vi "Init Array of VacuumLine Config Objs.vi"(8 "error in (no error)":errorcluster, 11 "VacuumLines Configuration in":refnum<class "VacuumLines Configuration.lvclass">) -> (0 "error out":errorcluster, 2 "Array of VacuumLine Config Objs":refnum<class "VacuumLine Configuration.lvclass">[](array[class]), 3 "VacuumLines Configuration out":refnum<class "VacuumLines Configuration.lvclass">)   [LabVIEW 2016, in "Hardware.lvlib" / "VacuumLine.lvlib" / "VacuumLines Configuration.lvclass"]
uses:
  <userlib>/Common Components/Hardware/Abstract System/VacuumLine/VacuumLines Configuration/VacuumLines Configuration.lvclass
  C:/Program Files (x86)/National Instruments/LabVIEW 2016/user.lib/Configuration Dialog Actor/Configuration.lvclass
  <userlib>/Common Components/Hardware/Abstract System/VacuumLine/VacuumLine Config/VacuumLine Configuration.lvclass
  <userlib>/Common Components/Hardware/Abstract System/VacuumLine/VacuumLines Configuration/VacuumLines Configuration.lvclass/VacuumLines Configuration.ctl
  <userlib>/Configuration Dialog Actor/Configuration.lvclass/Configuration.ctl
  <userlib>/Common Components/Hardware/Abstract System/VacuumLine/VacuumLines/VacuumLines.lvclass/VacuumLines.ctl
  <userlib>/Common Components/Hardware/Abstract System/VacuumLine/VacuumLine Config/VacuumLine Configuration.lvclass/VacuumLine Configuration.ctl
  <userlib>/Common Components/Hardware/Abstract System/VacuumLine/VacuumLine Config/Accessors/Write VacuumLine Obj.vi
  <userlib>/Configuration Dialog Actor/Accessors/Write Change Display.vi
  <userlib>/Configuration Dialog Actor/Accessors/Write Sub Panel.vi
  <userlib>/Configuration Dialog Actor/Accessors/Write Title.vi
  <userlib>/Configuration Dialog Actor/Accessors/Write Categories.vi
  <userlib>/Common Components/Hardware/Abstract System/VacuumLine/VacuumLines Configuration/Accessors/Read VacuumLines Obj.vi
  <userlib>/Configuration Dialog Actor/Accessors/Read Change Display.vi
  <userlib>/Configuration Dialog Actor/Accessors/Read Sub Panel.vi
  <userlib>/Configuration Dialog Actor/Accessors/Read Title.vi
  <userlib>/Configuration Dialog Actor/Accessors/Read Categories.vi
  <userlib>/Common Components/Hardware/Abstract System/VacuumLine/VacuumLines/VacuumLines.lvclass
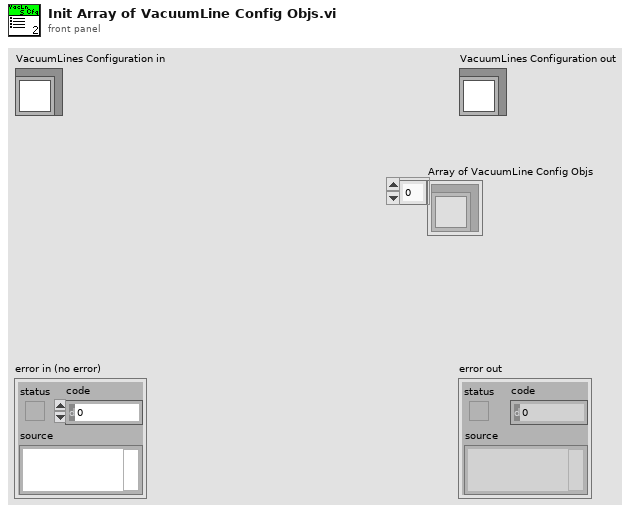
[diagram p1: front panel]
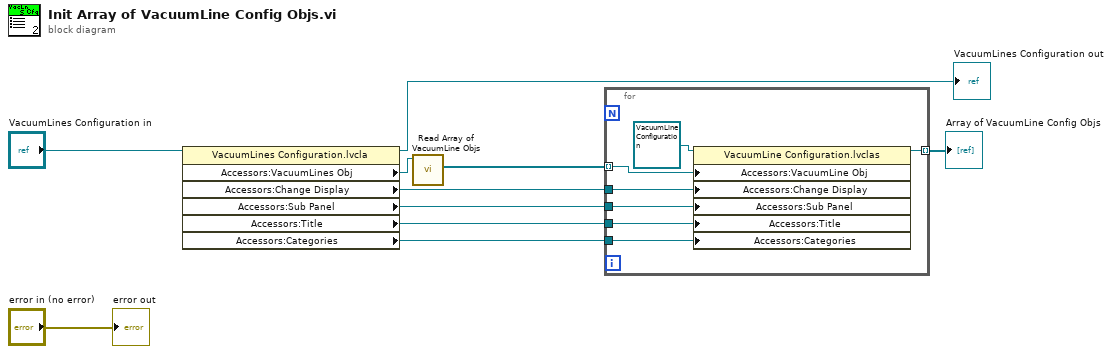
[diagram p0: block diagram]
diagram:
  n1 = property class="VacuumLines Configuration.lvcla"(reference="VacuumLines Configuration in") -> (reference out=→"VacuumLines Configuration out":refnum<class "VacuumLines Configuration.lvclass">, "Accessors:VacuumLines Obj"=w2:refnum<class "VacuumLines.lvclass">, "Accessors:Change Display"=w7:refnum<user-event>, "Accessors:Sub Panel"=w6:refnum<vi>, "Accessors:Title"=w5:refnum<vi>, "Accessors:Categories"=w4:refnum<vi>)  [unwired: 1 in, 1 out]
  n2 = call <userlib>:"Read Array of VacuumLine Objs.vi"("VacuumLines in"=w2) -> ("Array of VacuumLine Objs"=w1:refnum<class "VacuumLine.lvclass">[])  [unwired: 9 in, 1 out]
  n3 = for {
    tunnel: w7 -> [w17]
    tunnel: w6 -> [w16]
    tunnel: w5 -> [w15]
    tunnel: w4 -> [w14]
    tunnel: [w13] -> w3 mode=indexing
    tunnel: w1 -> [w11] mode=indexing
    n4 = property class="VacuumLine Configuration.lvclas"(reference=refnum<class "VacuumLine Configuration.lvclass"> refnum ("Hardware.lvlib:VacuumLine.lvlib:VacuumLine Configuration.lvclass"), "Accessors:VacuumLine Obj"=w11, "Accessors:Change Display"=w17, "Accessors:Sub Panel"=w16, "Accessors:Title"=w15, "Accessors:Categories"=w14) -> (reference out=w13:refnum<class "VacuumLine Configuration.lvclass">)  [unwired: 1 in, 1 out]
  }
  "Array of VacuumLine Config Objs" <- w3
  "error out" <- "error in (no error)"
